vi "Configure IF Gain (Others).vi"(8 "error in (no error)":errorcluster, 10 "IF Gain (0: Auto)":i32(ring) items=["Auto", "Low Gain", "High Gain"], 11 "VISA resource name":refnum<visa-resource-name>) -> (0 "error out":errorcluster, 3 "VISA resource name out":refnum<visa-resource-name>)   [LabVIEW 2018, in "Agilent MXA Series.lvlib"]
doc: "Configures the IF gain under Channel Power Measurement, Occupied Bandwith, Power Stat CCDF, ACP, Burst Power, Spurious Emissions and Spectrum Emission Mask measurement types."
uses:
  Agilent MXA Series.lvlib
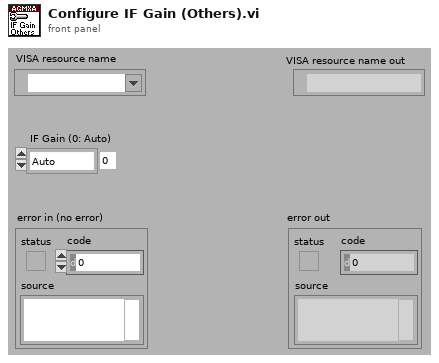
[diagram p1: front panel]
types:
  T1 = typedef "Agilent MXA Series.lvlib/Extended User Data.ctl" = cluster{"Measurement Type":i32, "Agilent MXA/EXA Model":i32}
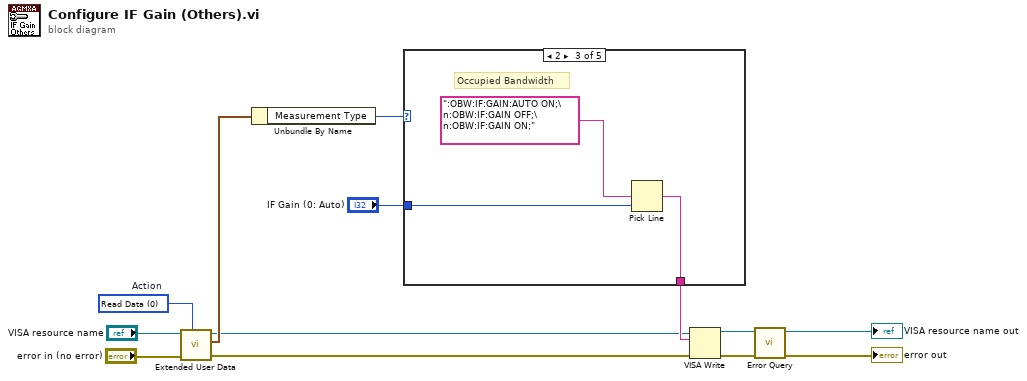
[diagram p0: block diagram]
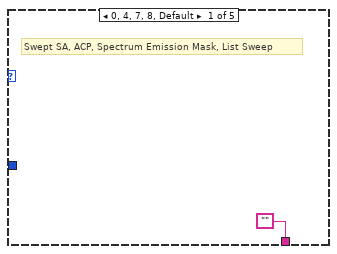
[diagram p2: hidden frame]
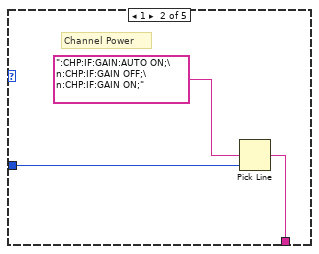
[diagram p3: hidden frame]
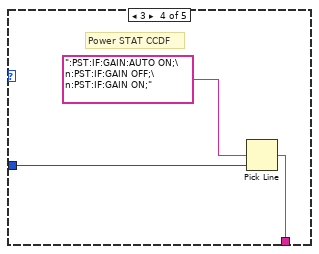
[diagram p4: hidden frame]
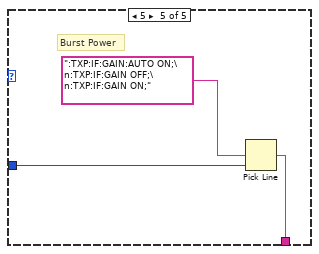
[diagram p5: hidden frame]
diagram:
  w11 = 0 items=["Read Data", "Write Data", "Clear Data", "Clear ALL Data"]  # Action
  n1 = call "Extended User Data.vi"("Action (1:Write Data)"=w11, "Error In (no error)"="error in (no error)", "VISA resource name in"="VISA resource name") -> ("Error Out"=w4:errorcluster, "User Data Out"=w10:T1, "VISA resource name out"=w6:refnum<visa-resource-name>)  [unwired: 6 in]
  n2 = Unbundle By Name(w10) -> ("Measurement Type"=w9:i32)
  n3 = case shown="2" w9 {
    tunnel: "IF Gain (0: Auto)" -> [_ w17 w19 w22 w25]
    tunnel: ["" w15 w18 w21 w24] -> w7
    frame 0, 4, 7, 8, Default {
      # "Swept SA, ACP, Spectrum Emission Mask, List Sweep"
    }
    frame 1 {
      # "Channel Power"
      n4 = Pick Line(multi-line string=":CHP:IF:GAIN:AUTO ON;\n:CHP:IF:GAIN OFF;\n:CHP:IF:GAIN ON;", line index=w17) -> (output string=w15:string)  [unwired: 1 in]
    }
    frame 2 {
      # "Occupied Bandwidth"
      n5 = Pick Line(multi-line string=":OBW:IF:GAIN:AUTO ON;\n:OBW:IF:GAIN OFF;\n:OBW:IF:GAIN ON;", line index=w19) -> (output string=w18:string)  [unwired: 1 in]
    }
    frame 3 {
      # "Power STAT CCDF"
      n6 = Pick Line(multi-line string=":PST:IF:GAIN:AUTO ON;\n:PST:IF:GAIN OFF;\n:PST:IF:GAIN ON;", line index=w22) -> (output string=w21:string)  [unwired: 1 in]
    }
    frame 5 {
      # "Burst Power"
      n7 = Pick Line(multi-line string=":TXP:IF:GAIN:AUTO ON;\n:TXP:IF:GAIN OFF;\n:TXP:IF:GAIN ON;", line index=w25) -> (output string=w24:string)  [unwired: 1 in]
    }
  }
  n8 = VISA Write(VISA resource name=w6, write buffer=w7, error in (no error)=w4) -> (VISA resource name out=w5:refnum<visa-resource-name>, error out=w3:errorcluster)  [unwired: 1 out]
  n9 = call "Error Query.vi"("error in (no error)"=w3, "VISA resource name"=w5) -> ("error out"=→"error out":errorcluster, "VISA resource name out"=→"VISA resource name out":refnum<visa-resource-name>)  [unwired: 6 in, 2 out]
